vi "secondUI_subVI.vi"(1 "Bool Refnum":refnum<vi>, 9 "Cluster1":refnum<vi>, 11 "Numeric":refnum<vi>, 12 "Stop Refnum":refnum<vi>) -> ()   [LabVIEW 2020]
panel:
  out "NewVal":T1
  out "Numeric":dbl
  out "Event Fired?":bool
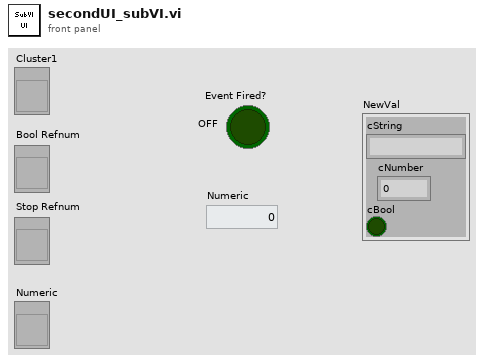
[diagram p1: front panel]
types:
  T1 = cluster{"cString":string, "cNumber":dbl, "cBool":bool}
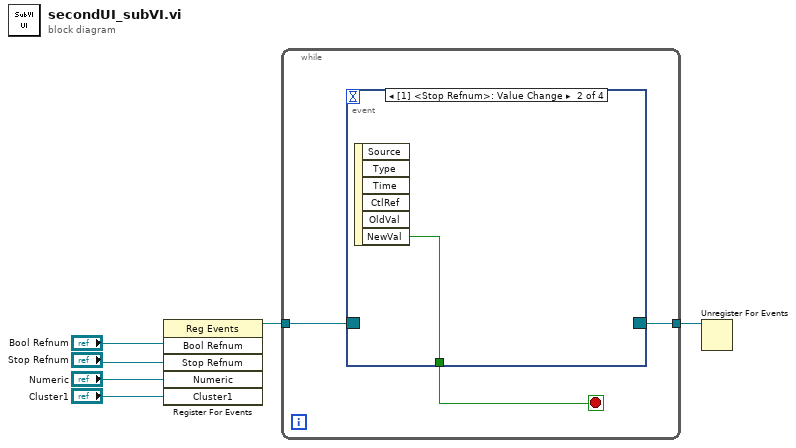
[diagram p0: block diagram]
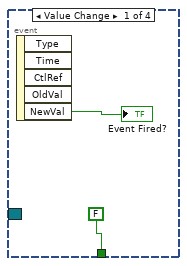
[diagram p2: hidden frame]
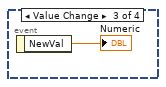
[diagram p3: hidden frame]
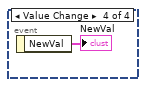
[diagram p4: hidden frame]
diagram:
  n1 = register-events("Bool Refnum", "Stop Refnum", "Numeric", "Cluster1") -> (reference out=w5:refnum<event-registration>)  [unwired: 2 in, 1 out]
  n2 = while {
    tunnel: w5 -> [w9]
    tunnel: [w7] -> w1
    stop <- w8 stop-if-true
    n3 = event shown="[1] <Stop Refnum>: Value Change" {
      selector: w9 -> [_ _ _ _]
      dyn-events: [_ _ _ _] -> w7
      timeout: _ -> [_ _ _ _]
      tunnel: [FALSE ("NewVal") w12 _ _] -> w8
      event Value Change {
        n4 = event-data() -> ("NewVal"=→"Event Fired?":bool)  [unwired: 1 in, 4 out]
      }
      event Value Change {
        n5 = event-data() -> ("NewVal"=w12:bool)  [unwired: 1 in, 5 out]
      }
      event Value Change {
        n6 = event-data() -> ("NewVal"=→"Numeric":dbl)  [unwired: 1 in]
      }
      event Value Change {
        n7 = event-data() -> ("NewVal"=→"NewVal":T1)  [unwired: 1 in]
      }
    }
  }
  n8 = Unregister For Events(event registration refnum=w1) -> ()  [unwired: 1 in, 1 out]
